vi "Plot new axis states.vi"(6 "GiveFocus?":bool, 9 "Multi-Y?":bool, 10 "Visible":bool, 11 "Scale LUT meta":T1) -> (2 "state change?":bool, 3 "Scale LUT meta":T1, 4 "Multi-y & no-focus":bool)   [LabVIEW 2021, in "RocketPlot.lvlib"]
uses:
  RocketPlot.lvlib
  TypeDefs/Plot scale meta JSON.ctl
  TypeDefs/Plot axis.ctl
  TypeDefs/Plot scale meta state.ctl
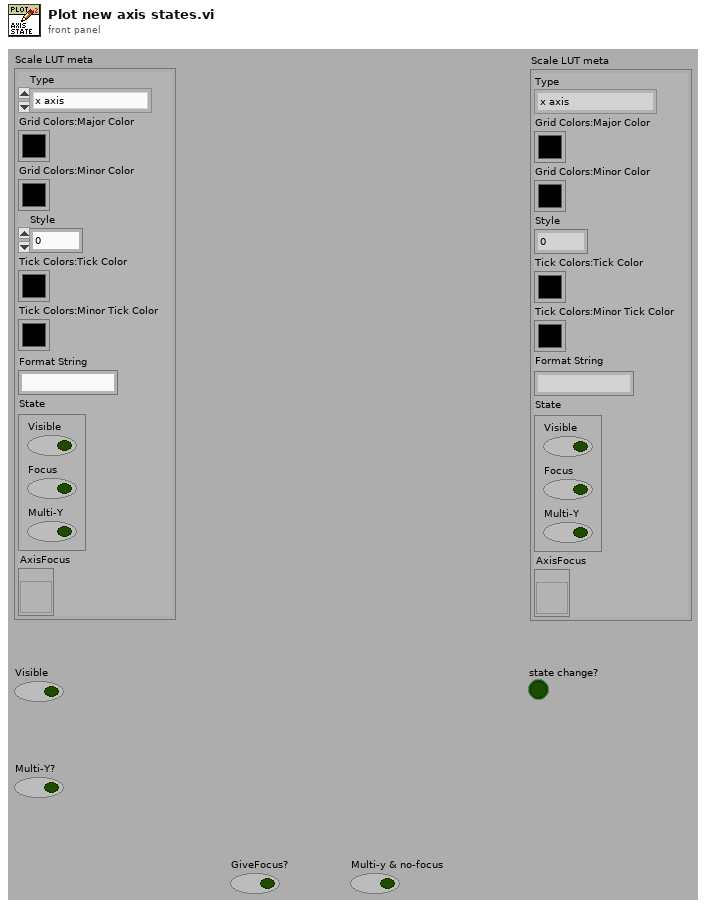
[diagram p1: front panel]
types:
  T1 = typedef "RocketPlot.lvlib/Plot scale meta JSON.ctl" = cluster{"Type":T2, "Grid Colors:Major Color":u32, "Grid Colors:Minor Color":u32, "Style":u8, "Tick Colors:Tick Color":u32, "Tick Colors:Minor Tick Color":u32, "Format String":string, "State":T3, "AxisFocus":refnum<vi>}
  T2 = typedef "RocketPlot.lvlib/Plot axis.ctl" = enum16{"x axis", "left axis", "right axis"}
  T3 = typedef "RocketPlot.lvlib/Plot scale meta state.ctl" = cluster{"Visible":bool, "Focus":bool, "Multi-Y":bool}
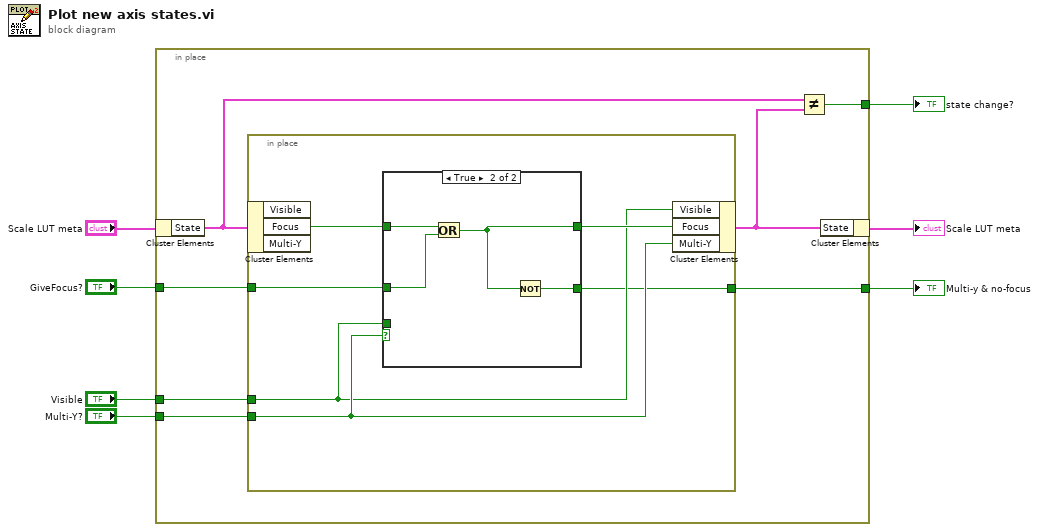
[diagram p0: block diagram]
diagram:
  n1 = in-place {
    in-place-border: "Visible" -> [w14]
    in-place-border: "Multi-Y?" -> [w13]
    in-place-border: [w11] -> w4
    in-place-border: [w9] -> w2
    in-place-border: "GiveFocus?" -> [w8]
    n2 = in-place-cluster #1("Scale LUT meta") -> ("State"=w12:T3)
    n3 = in-place {
      in-place-border: w14 -> [w17]
      in-place-border: w13 -> [w18]
      in-place-border: [w16] -> w9
      in-place-border: w8 -> [w15]
      n4 = in-place-cluster #2(w12) -> ("Focus"=w20:bool)  [unwired: 2 out]
      n5 = case shown="True" w18 {
        tunnel: w20 -> [_ w25]
        tunnel: [w21 w23] -> w19
        tunnel: w17 -> [w21 _]
        tunnel: [_ w22] -> w16
        tunnel: w15 -> [_ w24]
        frame False {
        }
        frame True {
          n6 = Or(x=w25, y=w24) -> (x .or. y?=w23:bool)
          n7 = Not(x=w23) -> (.not. x?=w22:bool)
        }
      }
      n8 = in-place-cluster #2("Visible"=w17, "Focus"=w19, "Multi-Y"=w18) -> (w10:T3)
    }
    n9 = Not Equal?(x=w12, y=w10) -> (x != y?=w11:bool)
    n10 = in-place-cluster #1("State"=w10) -> (→"Scale LUT meta":T1)
  }
  "state change?" <- w4
  "Multi-y & no-focus" <- w2
